vi "Build Channel Cluster Array.vi"(11 "Channels Amount":u8) -> (3 "Channels out":cluster{"Channels":T1[]})   [LabVIEW 2023, in "Device Cluster.lvclass"]
uses:
  Device Cluster.lvclass
  Utilities/Channel.ctl
  Device Cluster.lvclass/Device Cluster.ctl
  Utilities/Utilities.lvlib
panel:
  in  "Device Cluster.lvclass":refnum<class "Device Cluster.lvclass">
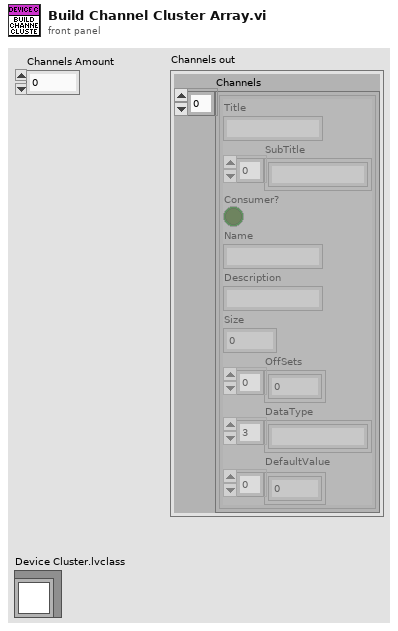
[diagram p1: front panel]
types:
  T1 = typedef "Utilities.lvlib/Channel.ctl" = cluster{"Title":string, "SubTitle":string[], "Consumer?":bool, "Name":string, "Description":string, "Size":i32, "OffSets":i32[], "DataType":string[], "DefaultValue":dbl[]}
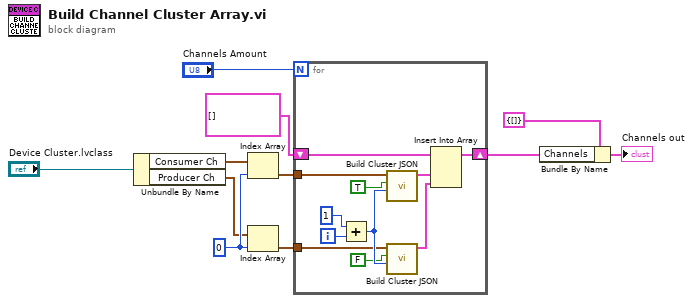
[diagram p0: block diagram]
diagram:
  w4 = 0 ("index")
  n1 = Unbundle By Name("Device Cluster.lvclass") -> ("Consumer Ch"=w6:cluster{"Voltage.SP":dbl, "Current.SP":dbl}[], "Producer Ch"=w3:cluster{"Voltage.AV":dbl, "Current.AV":dbl}[])
  n2 = Index Array(array=w6, index=w4) -> (element=w5:cluster{"Voltage.SP":dbl, "Current.SP":dbl})
  n3 = Index Array(array=w3, index=w4) -> (element=w2:cluster{"Voltage.AV":dbl, "Current.AV":dbl})
  n4 = for {
    N: "Channels Amount" -> [_]
    shift-right: [w18] -> w1
    shift-left: T1[] [] -> [w19]
    tunnel: w5 -> [w14]
    tunnel: w2 -> [w12]
    i -> [w17]
    n5 = Add(x=1, y=w17) -> (x+y=w15:i32)
    n6 = call "Build Cluster JSON.vi"("Channels Amount"=w15, "Consumer?"=TRUE, "Cluster"=w14) -> ("Array"=w21:T1[])  [unwired: 8 in]
    n7 = call "Build Cluster JSON.vi"("Channels Amount"=w15, "Consumer?"=FALSE, "Cluster"=w12) -> ("Array"=w20:T1[])  [unwired: 8 in]
    n8 = Insert Into Array(array=w19, new element #1=w21, new element #2=w20) -> (w18:T1[])  [unwired: 1 in]
  }
  n9 = Bundle By Name(cluster=cluster{"Channels":T1[]} {"Channels"=[]} ("Channels in"), "Channels"=w1) -> (→"Channels out":cluster{"Channels":T1[]})
